vi "DSF.Transceiver.UDP.Error.Create.vi"(9 "source vi name":string, 11 "Error":T1) -> (1 "offset":i32, 3 "error out":errorcluster)   [LabVIEW 2017, in "DSF.Transceiver.UDP.lvlib" / "DSF.Transceiver.UDP.lvclass"]
uses:
  DSF.Transceiver.UDP.lvclass
  DSF.Transceiver.UDP.Errors.ctl
  DSF.Transceiver.UDP.Constants.Library Name.vi
  <vilib>/NI/Static Error Handling/VIs/Static Error Handling.Error Cluster Constant (512B).vi
  <vilib>/NI/Static Error Handling/Static Error Handling.lvlib
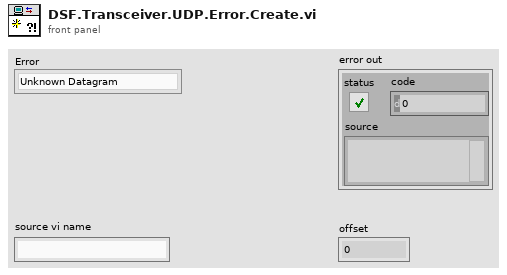
[diagram p1: front panel]
types:
  T1 = typedef "DSF.Transceiver.UDP.lvlib/DSF.Transceiver.UDP.lvclass/DSF.Transceiver.UDP.Errors.ctl" = enum16{"Unknown Datagram", "Size Mismatch"}
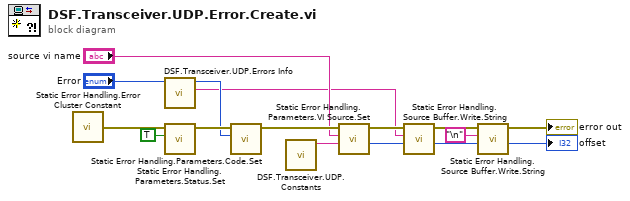
[diagram p0: block diagram]
diagram:
  n1 = call-poly <vilib>:"Static Error Handling.Error Cluster Constant.vi"() -> ("error out"=w15:errorcluster)  [unwired: 1 in]
  n2 = call "DSF.Transceiver.UDP.Errors Info.vi"("Error"="Error") -> ("description"=w6:string, "code"=w9:i32)  [unwired: 9 in]
  n3 = call <vilib>:"Static Error Handling.Parameters.Status.Set.vi"("status (T)"=TRUE, "error in"=w15) -> ("error out"=w13:errorcluster)  [unwired: 9 in]
  n4 = call <vilib>:"Static Error Handling.Parameters.Code.Set.vi"("code"=w9, "error in"=w13) -> ("error out"=w12:errorcluster)  [unwired: 9 in]
  n5 = call-poly "DSF.Transceiver.UDP.Constants.vi"() -> ("library name"=w10:string)  [unwired: 11 in]
  n6 = call <vilib>:"Static Error Handling.Parameters.VI Source.Set.vi"("library name (\"\")"=w10, "vi name"="source vi name", "error in"=w12) -> ("new offset"=w7:i32, "error out"=w8:errorcluster)  [unwired: 7 in]
  n7 = call <vilib>:"Static Error Handling.Source Buffer.Write.String.vi"("offset"=w7, "string"=w6, "error in"=w8) -> ("new offset"=w4:i32, "error out"=w5:errorcluster)  [unwired: 7 in]
  n8 = call <vilib>:"Static Error Handling.Source Buffer.Write.String.vi"("offset"=w4, "string"="\n", "error in"=w5) -> ("new offset"=→"offset":i32, "error out"=→"error out":errorcluster)  [unwired: 7 in]
